vi "MCS_AutoZero.vi"(1 "error in (no error)":errorcluster, 2 "System Index In":u32) -> (0 "error out":errorcluster)   [LabVIEW 2010]
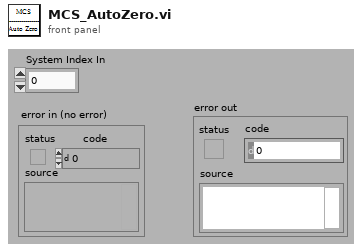
[diagram p1: front panel]
types:
  T1 = enum32{"SA_FORWARD_DIRECTION", "SA_BACKWARD_DIRECTION", "SA_FORWARD_BACKWARD_DIRECTION", "SA_BACKWARD_FORWARD_DIRECTION"}
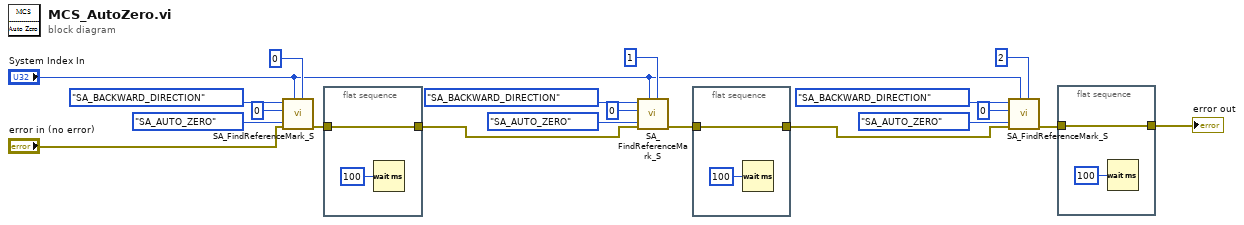
[diagram p0: block diagram]
diagram:
  n1 = call <vilib>:"SA_FindReferenceMark_S.vi"("channelIndex"=u32 0, "systemIndex"="System Index In", "error in (no error)"="error in (no error)", "autoZero"=enum32{"SA_NO_AUTO_ZERO", "SA_AUTO_ZERO"}."SA_AUTO_ZERO", "holdTime"=u32 0, "direction"=T1."SA_BACKWARD_DIRECTION") -> ("error out"=w11:errorcluster)  [unwired: 5 in]
  n2 = flat-sequence {
    tunnel: w11 -> [w21]
    tunnel: [w21] -> w10
    frame #0 {
      n3 = Wait (ms)(milliseconds to wait=u32 100) -> ()  [unwired: 1 out]
    }
  }
  n4 = call <vilib>:"SA_FindReferenceMark_S.vi"("channelIndex"=u32 1, "systemIndex"="System Index In", "error in (no error)"=w10, "autoZero"=enum32{"SA_NO_AUTO_ZERO", "SA_AUTO_ZERO"}."SA_AUTO_ZERO", "holdTime"=u32 0, "direction"=T1."SA_BACKWARD_DIRECTION") -> ("error out"=w4:errorcluster)  [unwired: 5 in]
  n5 = flat-sequence {
    tunnel: w4 -> [w23]
    tunnel: [w23] -> w5
    frame #0 {
      n6 = Wait (ms)(milliseconds to wait=u32 100) -> ()  [unwired: 1 out]
    }
  }
  n7 = call <vilib>:"SA_FindReferenceMark_S.vi"("channelIndex"=u32 2, "systemIndex"="System Index In", "error in (no error)"=w5, "autoZero"=enum32{"SA_NO_AUTO_ZERO", "SA_AUTO_ZERO"}."SA_AUTO_ZERO", "holdTime"=u32 0, "direction"=T1."SA_BACKWARD_DIRECTION") -> ("error out"=w3:errorcluster)  [unwired: 5 in]
  n8 = flat-sequence {
    tunnel: w3 -> [w25]
    tunnel: [w25] -> w1
    frame #0 {
      n9 = Wait (ms)(milliseconds to wait=u32 100) -> ()  [unwired: 1 out]
    }
  }
  "error out" <- w1
